vi "FL_Filter_data_for_online_display.vi"(3 "Input data":cluster{"X1":dbl, "Y1":dbl, "X2":dbl, "Y2":dbl}, 4 "Filter type":u16(ring)=5 items=["None", "Kalman 0.50", "Kalman 0.30", "Kalman 0.12", "Savitzky-Golay 3/5", "Savitzky-Golay 3/11", "Savitzky-Golay 3/31"], 5 "Data filtered on previous step":cluster{"X1":dbl, "Y1":dbl, "X2":dbl, "Y2":dbl}) -> (1 "Output data":cluster{"X1":dbl, "Y1":dbl, "X2":dbl, "Y2":dbl})   [LabVIEW 2016]
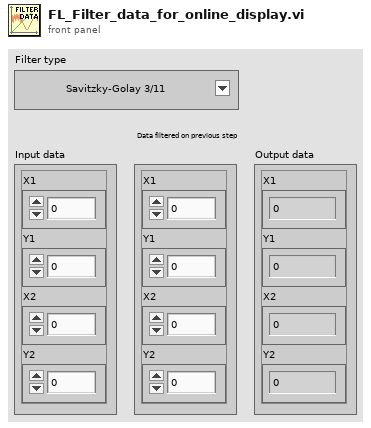
[diagram p1: front panel]
types:
  T1 = cluster{"[0]":dbl, "[1]":dbl, "[2]":dbl, "[3]":dbl}
  T2 = cluster{"0th order SG coefficients":dbl[], "1st order SG coefficients":dbl[]}
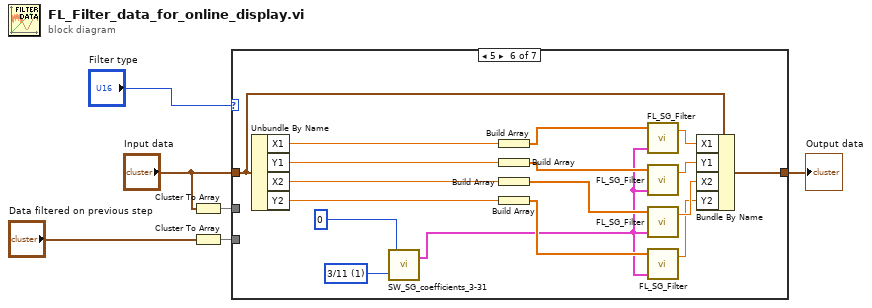
[diagram p0: block diagram]
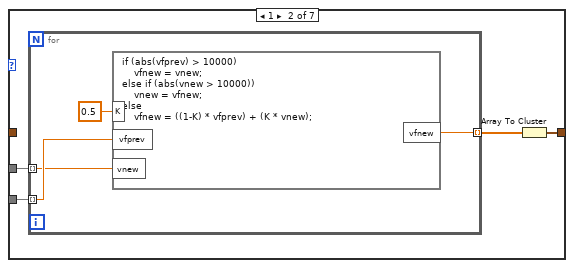
[diagram p3: hidden frame]
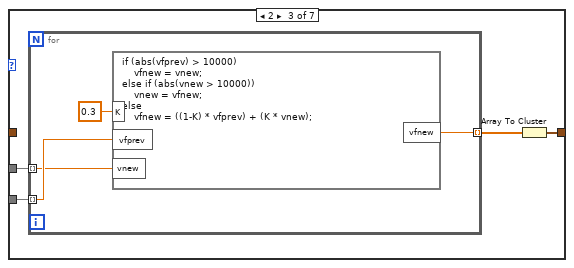
[diagram p4: hidden frame]
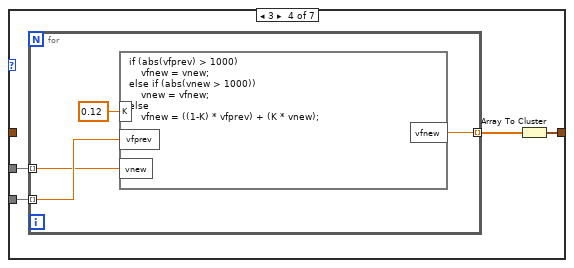
[diagram p5: hidden frame]
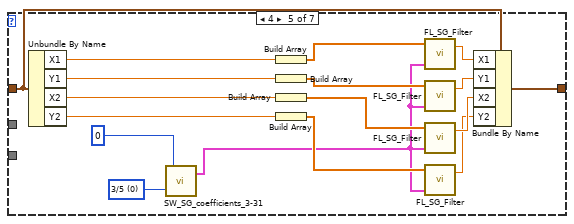
[diagram p6: hidden frame]
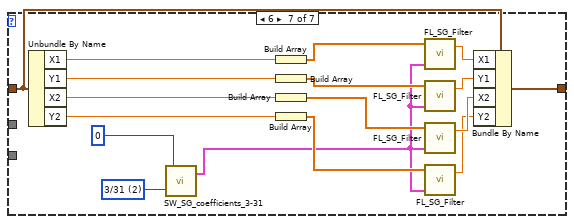
[diagram p7: hidden frame]
diagram:
  n1 = Cluster To Array(cluster="Input data") -> (array=w3:dbl[])
  n2 = Cluster To Array(cluster="Data filtered on previous step") -> (array=w5:dbl[])
  n3 = case shown="5" "Filter type" {
    tunnel: w5 -> [_ w11 w19 w27 _ _ _]
    tunnel: [w7 w9 w17 w25 w35 w52 w69] -> w4
    tunnel: w3 -> [_ w8 w16 w24 _ _ _]
    tunnel: "Input data" -> [w7 _ _ _ w40 w57 w74]
    frame 0, Default {
    }
    frame 1 {
      n4 = for {
        tunnel: w8 -> [w14] mode=indexing
        tunnel: w11 -> [w15] mode=indexing
        tunnel: [w13] -> w10 mode=indexing
        n5 = formula code="if (abs(vfprev) > 10000)\n    vfnew = vnew;\nelse if (abs(vnew > 10000))\n    vnew = vfnew;\nelse\n    vfnew = ((1-K) * vfprev) + (K * vnew);"("K"=0.5 ("input variable"), "vfprev"=w15, "vnew"=w14) -> ("vfnew"=w13:dbl)
      }
      n6 = Array To Cluster(array=w10) -> (cluster=w9:T1)
    }
    frame 2 {
      n7 = for {
        tunnel: w16 -> [w22] mode=indexing
        tunnel: w19 -> [w23] mode=indexing
        tunnel: [w21] -> w18 mode=indexing
        n8 = formula code="if (abs(vfprev) > 10000)\n    vfnew = vnew;\nelse if (abs(vnew > 10000))\n    vnew = vfnew;\nelse\n    vfnew = ((1-K) * vfprev) + (K * vnew);"("K"=0.3 ("input variable"), "vfprev"=w23, "vnew"=w22) -> ("vfnew"=w21:dbl)
      }
      n9 = Array To Cluster(array=w18) -> (cluster=w17:T1)
    }
    frame 3 {
      n10 = for {
        tunnel: w24 -> [w30] mode=indexing
        tunnel: w27 -> [w31] mode=indexing
        tunnel: [w29] -> w26 mode=indexing
        n11 = formula code="if (abs(vfprev) > 1000)\n    vfnew = vnew;\nelse if (abs(vnew > 1000))\n    vnew = vfnew;\nelse\n    vfnew = ((1-K) * vfprev) + (K * vnew);"("K"=0.12 ("input variable"), "vfprev"=w31, "vnew"=w30) -> ("vfnew"=w29:dbl)
      }
      n12 = Array To Cluster(array=w26) -> (cluster=w25:T1)
    }
    frame 4 {
      w32 = u16 0 items=["3/5", "3/11", "3/31"] ("Select filter length")
      n13 = Unbundle By Name(w40) -> ("X1"=w47:dbl, "Y1"=w45:dbl, "X2"=w44:dbl, "Y2"=w43:dbl)
      n14 = call "SW_SG_coefficients_3-31.vi"("Select filter length"=w32, "Point of interest (can be used for extrapolation)"=0) -> ("SG coefficients"=w34:T2)  [unwired: 1 in]
      n15 = Build Array(w47) -> (w48:dbl[])
      n16 = Build Array(w45) -> (w46:dbl[])
      n17 = Build Array(w44) -> (w42:dbl[])
      n18 = Build Array(w43) -> (w41:dbl[])
      n19 = call "FL_SG_Filter.vi"("SG coefficients"=w34, "Input array of data"=w48) -> ("Filtered data, 0 order"=w39:dbl)  [unwired: 2 in]
      n20 = call "FL_SG_Filter.vi"("SG coefficients"=w34, "Input array of data"=w46) -> ("Filtered data, 0 order"=w38:dbl)  [unwired: 2 in]
      n21 = call "FL_SG_Filter.vi"("SG coefficients"=w34, "Input array of data"=w42) -> ("Filtered data, 0 order"=w37:dbl)  [unwired: 2 in]
      n22 = call "FL_SG_Filter.vi"("SG coefficients"=w34, "Input array of data"=w41) -> ("Filtered data, 0 order"=w36:dbl)  [unwired: 2 in]
      n23 = Bundle By Name(cluster=w40, "X1"=w39, "Y1"=w38, "X2"=w37, "Y2"=w36) -> (w35:cluster{"X1":dbl, "Y1":dbl, "X2":dbl, "Y2":dbl})
    }
    frame 5 {
      w49 = u16 1 items=["3/5", "3/11", "3/31"] ("Select filter length")
      n24 = Unbundle By Name(w57) -> ("X1"=w64:dbl, "Y1"=w62:dbl, "X2"=w61:dbl, "Y2"=w60:dbl)
      n25 = call "SW_SG_coefficients_3-31.vi"("Select filter length"=w49, "Point of interest (can be used for extrapolation)"=0) -> ("SG coefficients"=w51:T2)  [unwired: 1 in]
      n26 = Build Array(w64) -> (w65:dbl[])
      n27 = Build Array(w62) -> (w63:dbl[])
      n28 = Build Array(w61) -> (w59:dbl[])
      n29 = Build Array(w60) -> (w58:dbl[])
      n30 = call "FL_SG_Filter.vi"("SG coefficients"=w51, "Input array of data"=w65) -> ("Filtered data, 0 order"=w56:dbl)  [unwired: 2 in]
      n31 = call "FL_SG_Filter.vi"("SG coefficients"=w51, "Input array of data"=w63) -> ("Filtered data, 0 order"=w55:dbl)  [unwired: 2 in]
      n32 = call "FL_SG_Filter.vi"("SG coefficients"=w51, "Input array of data"=w59) -> ("Filtered data, 0 order"=w54:dbl)  [unwired: 2 in]
      n33 = call "FL_SG_Filter.vi"("SG coefficients"=w51, "Input array of data"=w58) -> ("Filtered data, 0 order"=w53:dbl)  [unwired: 2 in]
      n34 = Bundle By Name(cluster=w57, "X1"=w56, "Y1"=w55, "X2"=w54, "Y2"=w53) -> (w52:cluster{"X1":dbl, "Y1":dbl, "X2":dbl, "Y2":dbl})
    }
    frame 6 {
      w66 = u16 2 items=["3/5", "3/11", "3/31"] ("Select filter length")
      n35 = Unbundle By Name(w74) -> ("X1"=w81:dbl, "Y1"=w79:dbl, "X2"=w78:dbl, "Y2"=w77:dbl)
      n36 = call "SW_SG_coefficients_3-31.vi"("Select filter length"=w66, "Point of interest (can be used for extrapolation)"=0) -> ("SG coefficients"=w68:T2)  [unwired: 1 in]
      n37 = Build Array(w81) -> (w82:dbl[])
      n38 = Build Array(w79) -> (w80:dbl[])
      n39 = Build Array(w78) -> (w76:dbl[])
      n40 = Build Array(w77) -> (w75:dbl[])
      n41 = call "FL_SG_Filter.vi"("SG coefficients"=w68, "Input array of data"=w82) -> ("Filtered data, 0 order"=w73:dbl)  [unwired: 2 in]
      n42 = call "FL_SG_Filter.vi"("SG coefficients"=w68, "Input array of data"=w80) -> ("Filtered data, 0 order"=w72:dbl)  [unwired: 2 in]
      n43 = call "FL_SG_Filter.vi"("SG coefficients"=w68, "Input array of data"=w76) -> ("Filtered data, 0 order"=w71:dbl)  [unwired: 2 in]
      n44 = call "FL_SG_Filter.vi"("SG coefficients"=w68, "Input array of data"=w75) -> ("Filtered data, 0 order"=w70:dbl)  [unwired: 2 in]
      n45 = Bundle By Name(cluster=w74, "X1"=w73, "Y1"=w72, "X2"=w71, "Y2"=w70) -> (w69:cluster{"X1":dbl, "Y1":dbl, "X2":dbl, "Y2":dbl})
    }
  }
  "Output data" <- w4
